vi "gfitsio-check-image-for-write.vi"(4 "lpixel":i32[](array[numeric]), 6 "fpixel":i32[](array[numeric]), 8 "error in (no error)":errorcluster, 11 "gfits refnum":T1) -> (0 "error out":errorcluster, 3 "dup gfits refnum":T1)   [LabVIEW 2011, in "gfitsio.lvlib"]
uses:
  gfitsio.lvlib
  gfitsio-refnum.ctl
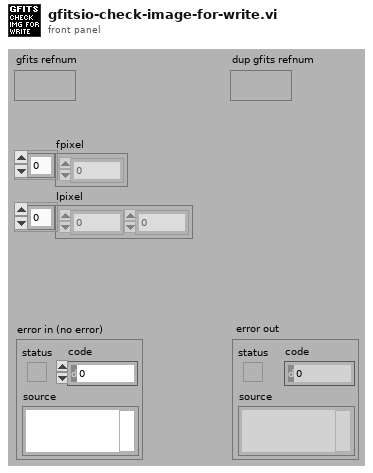
[diagram p1: front panel]
types:
  T1 = typedef "gfitsio.lvlib/gfitsio-refnum.ctl" = refnum<k1>
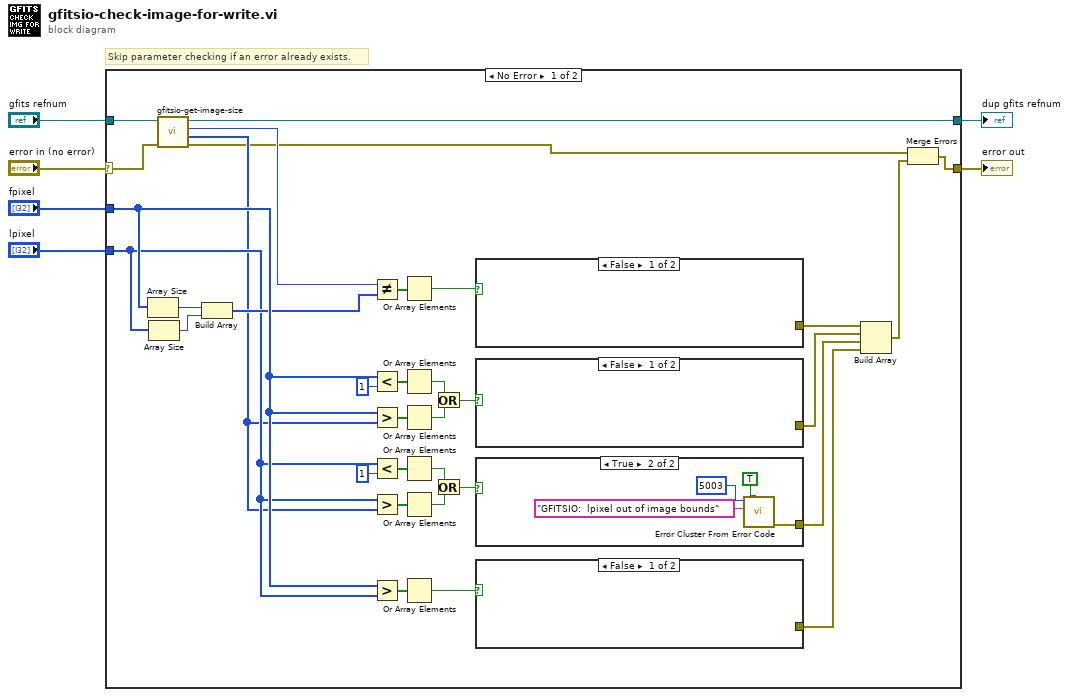
[diagram p0: block diagram]
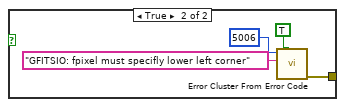
[diagram p2: hidden frame]
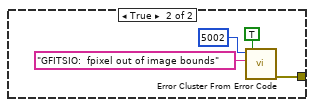
[diagram p4: hidden frame]
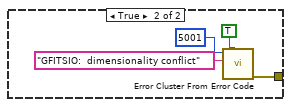
[diagram p5: hidden frame]
diagram:
  # "Skip parameter checking if an error already exists."
  n1 = case shown="No Error" "error in (no error)" {
    selector: "error in (no error)" -> [w38 w57]
    tunnel: "gfits refnum" -> [w39 w56]
    tunnel: [w7 w56] -> w2
    tunnel: "fpixel" -> [w17 _]
    tunnel: "lpixel" -> [w10 _]
    tunnel: [w37 w57] -> w6
    frame No Error {
      n2 = Array Size(array=w17) -> (size(s)=w16:i32)
      n3 = Array Size(array=w10) -> (size(s)=w15:i32)
      n4 = call "gfitsio-get-image-size.vi"("error in (no error)"=w38, "gfits refnum"=w39) -> ("error out"=w8:errorcluster, "naxes"=w9:i32[], "naxis"=w34:i32, "dup gfits refnum"=w7:T1)  [unwired: 6 in]
      n5 = Build Array(w16, w15) -> (w14:i32[])
      n6 = Not Equal?(x=w34, y=w14) -> (x != y?=w13:bool[])
      n7 = Less?(x=w17, y=1 ("x")) -> (x < y?=w30:bool[])
      n8 = Greater?(x=w17, y=w9) -> (0:w29:bool[])
      n9 = Less?(x=w10, y=1 ("x")) -> (x < y?=w22:bool[])
      n10 = Greater?(x=w10, y=w9) -> (0:w23:bool[])
      n11 = Greater?(x=w17, y=w10) -> (0:w19:bool[])
      n12 = Or Array Elements(Boolean array=w13) -> (logical OR=w12:bool)
      n13 = Or Array Elements(Boolean array=w30) -> (logical OR=w27:bool)
      n14 = Or Array Elements(Boolean array=w29) -> (logical OR=w26:bool)
      n15 = Or Array Elements(Boolean array=w22) -> (logical OR=w24:bool)
      n16 = Or Array Elements(Boolean array=w23) -> (logical OR=w25:bool)
      n17 = Or Array Elements(Boolean array=w19) -> (logical OR=w18:bool)
      n18 = Or(x=w27, y=w26) -> (x .or. y?=w28:bool)
      n19 = Or(x=w24, y=w25) -> (x .or. y?=w20:bool)
      n20 = case shown="False" w12 {
        tunnel: [_ w53] -> w36
        frame False {
        }
        frame True {
          n21 = call <vilib>:"Error Cluster From Error Code.vi"("show call chain? (False)"=TRUE, "error message (\"\")"="GFITSIO:  dimensionality conflict" ("error message (\"\")"), "error code (0)"=5001) -> ("error out"=w53:errorcluster)  [unwired: 6 in]
        }
      }
      n22 = case shown="False" w28 {
        tunnel: [_ w49] -> w33
        frame False {
        }
        frame True {
          n23 = call <vilib>:"Error Cluster From Error Code.vi"("show call chain? (False)"=TRUE, "error message (\"\")"="GFITSIO:  fpixel out of image bounds" ("error message (\"\")"), "error code (0)"=5002) -> ("error out"=w49:errorcluster)  [unwired: 6 in]
        }
      }
      n24 = case shown="True" w20 {
        tunnel: [_ w45] -> w32
        frame False {
        }
        frame True {
          n25 = call <vilib>:"Error Cluster From Error Code.vi"("show call chain? (False)"=TRUE, "error message (\"\")"="GFITSIO:  lpixel out of image bounds" ("error message (\"\")"), "error code (0)"=5003) -> ("error out"=w45:errorcluster)  [unwired: 6 in]
        }
      }
      n26 = case shown="False" w18 {
        tunnel: [_ w41] -> w11
        frame False {
        }
        frame True {
          n27 = call <vilib>:"Error Cluster From Error Code.vi"("show call chain? (False)"=TRUE, "error message (\"\")"="GFITSIO: fpixel must specifly lower left corner" ("error message (\"\")"), "error code (0)"=5006) -> ("error out"=w41:errorcluster)  [unwired: 6 in]
        }
      }
      n28 = Build Array(w36, w33, w32, w11) -> (w35:errorcluster[])
      n29 = Merge Errors(w8, w35) -> (w37:errorcluster)
    }
    frame Error {
    }
  }
  "error out" <- w6
  "dup gfits refnum" <- w2
